vi "Winch.vi"(10 "setpoint":dbl format="%.2f") -> (2 "Actual":dbl format="%#_13g")   [LabVIEW 2013]
uses:
  <vilib>/Rock Robotics/WPI/SafetyOutput/WPI_SafetyOutputConfigMenu.ctl
  Begin/Global Refnums.vi
  <vilib>/addons/control/pid/pid.llb/PID (DBL).vi
  <vilib>/addons/control/pid/NI_PID_pid.lvlib
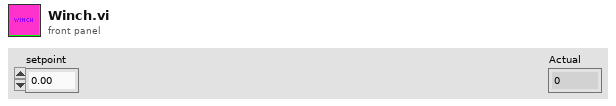
[diagram p1: front panel]
types:
  T1 = typedef "WPI_SafetyOutputConfigMenu.ctl" = enum16{"Enable", "Disable"}
  T2 = cluster{"proportional gain (Kc)":dbl, "integral time (Ti, min)":dbl, "derivative time (Td, min)":dbl}
  T3 = typedef "WPI_AnalogChannelDevRef.ctl" = cluster{"DevStatus":errorcluster, "Analog Module":T4, "Analog Channel":T5}
  T4 = typedef "FPGA_TypedefAnalogModule.ctl" = enum16{"Analog Module 1", "Analog Module 2"}
  T5 = typedef "FPGA_AIChannel.ctl" = enum8{"AI 1", "AI 2", "AI 3", "AI 4", "AI 5", "AI 6", "AI 7", "AI 8", "Invalid"}
  T6 = typedef "WPI_MotorControlDeviceRef.ctl" = cluster{"DeviceStatus":errorcluster, "Type":enum16{"PWM", "CAN"}, "PWM":cluster{"Digital Module":T7, "PWM Channel":T8, "DeadBand":T9}, "CAN":cluster{"Device Number":u8, "Control Mode":T10, "Semaphore":T11, "Max Vout":dbl}, "Invert":bool, "TransformRef":T12, "InvTransformRef":T12}
  T7 = typedef "FPGA_TypedefDigitalModule.ctl" = enum16{"Digital Module 1", "Digital Module 2"}
  T8 = typedef "FPGA_DIOPWMChannel.ctl" = enum8{"PWM 1", "PWM 2", "PWM 3", "PWM 4", "PWM 5", "PWM 6", "PWM 7", "PWM 8", "PWM 9", "PWM 10", "Invalid"}
  T9 = typedef "WPI_PWMDeadband.ctl" = cluster{"Name":string, "maxPositivePwm":i32, "minPositivePwm":i32, "centerPwm":i32, "maxNegativePwm":i32, "minNegativePwm":i32, "angularRange":u16}
  T10 = typedef "WPI_CANJaguar_ControlMode.ctl" = enum8{"Percent VBus", "Current", "Speed", "Position", "Voltage"}
  T11 = typedef "Semaphore RefNum" = refnum<k1>
  T12 = typedef "WPI_PWMTransform_ConPane.ctl" = refnum<vi>
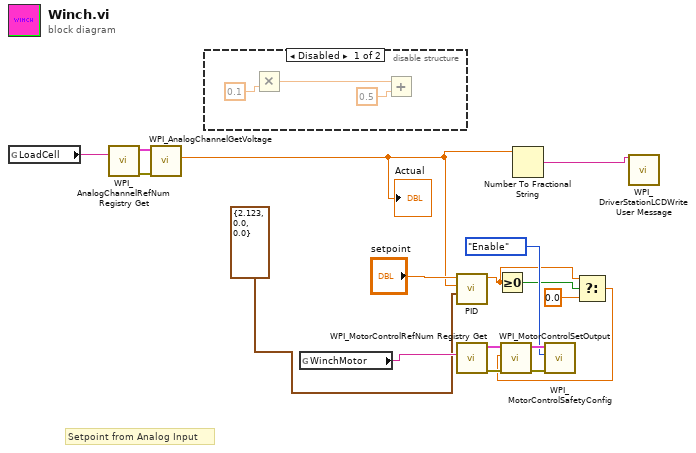
[diagram p0: block diagram]
diagram:
  # "Setpoint from Analog Input"
  n1 = global read "Global Refnums.vi" "LoadCell"() -> (w6:string)
  n2 = call <vilib>:"WPI_AnalogChannelRefNum Registry Get.vi"("refnum name"=w6) -> ("error out"=w11:errorcluster, "AIDeviceRef"=w12:T3)  [unwired: 9 in]
  n3 = call <vilib>:"WPI_AnalogChannelGetVoltage.vi"("error in (no error)"=w11, "AIDeviceRef"=w12) -> ("Voltage"=w1:dbl)  [unwired: 7 in, 2 out]
  "Actual" <- w1
  n4 = disable-structure shown="Disabled" {
    frame Disabled {
      n5 = Multiply(y=0.1) -> (x*y=w19:dbl)  [unwired: 1 in]
      n6 = Add(x=w19, y=0.5) -> ()  [unwired: 1 out]
    }
    frame Enabled {
    }
  }
  n7 = global read "Global Refnums.vi" "WinchMotor"() -> (w5:string)
  n8 = call-poly <vilib>:"PID.vi"("PID gains"=T2 {"proportional gain (Kc)"=2.123, "integral time (Ti, min)"=0.0, "derivative time (Td, min)"=0.0}, "process variable"=w1, "setpoint"="setpoint") -> ("output"=w9:dbl)  [unwired: 7 in, 1 out]
  n9 = call <vilib>:"WPI_MotorControlRefNum Registry Get.vi"("refnum name"=w5) -> ("error out"=w13:errorcluster, "MotorControlDevRef"=w14:T6)  [unwired: 9 in]
  n10 = Greater Or Equal To 0?(x=w9) -> (x >= 0?=w10:bool)
  n11 = Number To Fractional String(number=w1) -> (F-format string=w4:string)  [unwired: 3 in]
  n12 = Select(t=w9, s=w10, f=0.0) -> (s? t:f=w8:dbl)
  n13 = call <vilib>:"WPI_MotorControlSetOutput.vi"("error in (no error)"=w13, "Output"=w8, "MotorControlDevRef"=w14) -> ("error out"=w15:errorcluster, "MotorControlDevRef"=w17:T6)  [unwired: 6 in, 1 out]
  n14 = call <vilib>:"WPI_MotorControlSafetyConfig.vi"("error in (no error)"=w15, "mode"=WPI_SafetyOutputConfigMenu."Enable", "MotorControlDevRef"=w17) -> ()  [unwired: 7 in, 2 out]
  n15 = call <vilib>:"WPI_DriverStationLCDWrite User Message.vi"("line text"=w4) -> ()  [unwired: 14 in, 1 out]
